vi "GetType.vi"(8 "error in (no error)":errorcluster, 11 "Configure Internal Trigger Rate [IT] Msg in":refnum<class "Configure Internal Trigger Rate [IT] Msg.lvclass">) -> (0 "error out":errorcluster, 2 "Data Sample":variant, 3 "Configure Internal Trigger Rate [IT] Msg out":refnum<class "Configure Internal Trigger Rate [IT] Msg.lvclass">)   [LabVIEW 2014, in "CS++Fgen.lvlib" / "Configure Internal Trigger Rate [IT] Msg.lvclass"]
doc: "This VI delivers a sample of the data type format the message expects."
uses:
  Configure Internal Trigger Rate [IT] Msg.lvclass
  Configure Internal Trigger Rate [IT] Msg.lvclass/Configure Internal Trigger Rate [IT] Msg.ctl
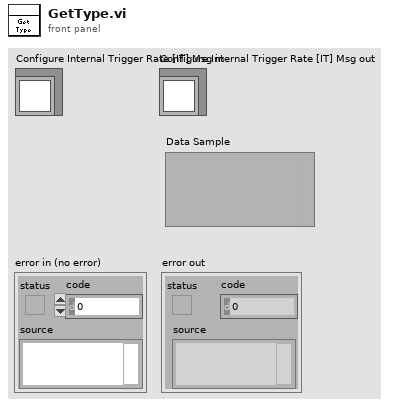
[diagram p1: front panel]
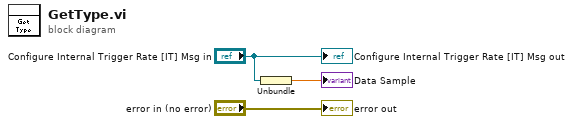
[diagram p0: block diagram]
diagram:
  n1 = Unbundle("Configure Internal Trigger Rate [IT] Msg in") -> (→"Data Sample":dbl[unit])
  "error out" <- "error in (no error)"
  "Configure Internal Trigger Rate [IT] Msg out" <- "Configure Internal Trigger Rate [IT] Msg in"
